vi "DestroyPublicEvents.vi"(8 "error in (no error)":errorcluster, 11 "SMO.Dictionary":refnum<class "SMO.Dictionary.lvclass">) -> (0 "error out":errorcluster, 3 "SMO.Dictionary out":refnum<class "SMO.Dictionary.lvclass">)   [LabVIEW 2013, in "SMO.Dictionary.lvlib" / "SMO.Dictionary.lvclass"]
doc: "JKI State Machine Objects (SMO) 1.0.1.12\nJKI - JKI\nCopyright (c) 2016, JKI"
uses:
  SMO.Dictionary.lvclass
  <vilib>/JKI/JKI SMO/SMO/SMO.lvclass
panel:
  # "For instructions on how to use the JKI State Machine Objects, examples and video tutorials, visit:\nhttp://jki.net/state-machine-objects/\n\nJKI State Machine Objects™\nhttp://jki.net/state-machine-objects/\nCopyright (C) 2005-2015, JKI <info@jki.net>\nALL RIGHTS RESERVED"
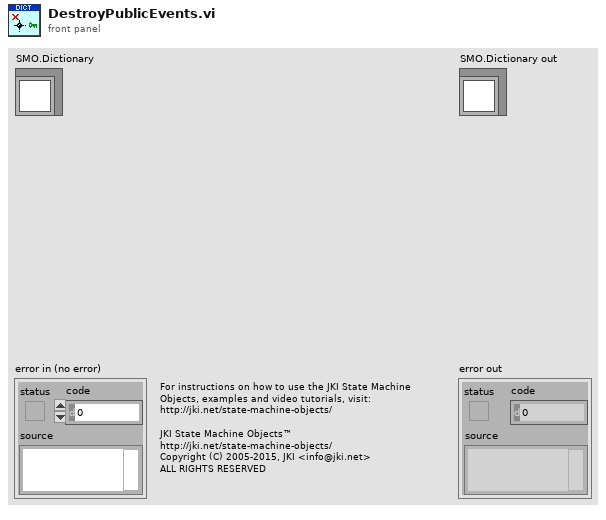
[diagram p1: front panel]
types:
  T1 = typedef "SMO.Dictionary.lvlib/SMO.Dictionary.lvclass/PublicEvents--Cluster.ctl" = cluster{"Cleared":refnum<user-event>, "Deleted":refnum<user-event>, "Updated":refnum<user-event>}
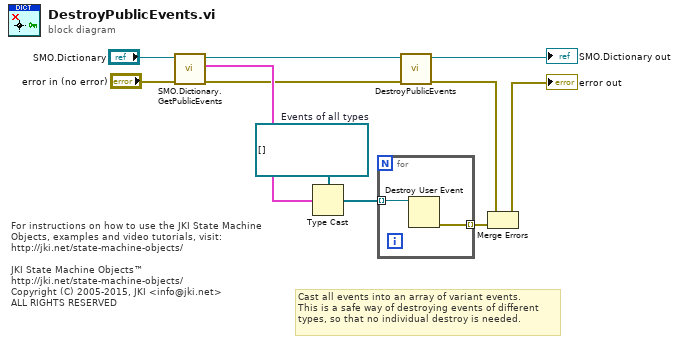
[diagram p0: block diagram]
diagram:
  w9 = refnum<user-event>[] []  # Events of all types
  # "For instructions on how to use the JKI State Machine Objects, examples and video tutorials, visit:\nhttp://jki.net/state-machine-objects/\n\nJKI State Machine Objects™\nhttp://jki.net/state-machine-objects/\nCopyright (C) 2005-2015, JKI <info@jki.net>\nALL RIGHTS RESERVED"
  # "Cast all events into an array of variant events.\nThis is a safe way of destroying events of different\ntypes, so that no individual destroy is needed."
  n1 = call "SMO.Dictionary.GetPublicEvents.vi"("error in (no error)"="error in (no error)", "SMO.Dictionary in"="SMO.Dictionary") -> ("error out"=w3:errorcluster, "Public Events"=w6:T1, "SMO.Dictionary out"=w5:refnum<class "SMO.Dictionary.lvclass">)  [unwired: 7 in]
  n2 = Type Cast(type=w9, x=w6) -> (*(type *) &x=w10:refnum<user-event>[])
  n3 = for {
    tunnel: w10 -> [w13] mode=indexing
    tunnel: [w12] -> w8 mode=indexing
    n4 = Destroy User Event(user event=w13) -> (error out=w12:errorcluster)  [unwired: 1 in]
  }
  n5 = call-parent "DestroyPublicEvents.vi"("error in (no error)"=w3, "SMO"=w5) -> ("error out"=w11:errorcluster, "SMO out"=→"SMO.Dictionary out":refnum<class "SMO.Dictionary.lvclass">)  [unwired: 8 in]
  n6 = Merge Errors(w11, w8) -> (→"error out":errorcluster)
